vi "sub_ofdm_mes_ce.vi"(11 "ZF channel estimates":cdb[](array[numeric])) -> (3 "interpolated mes carrier CE":cdb[](array[numeric]))   [LabVIEW 2014]
panel:
  out "output size":i32
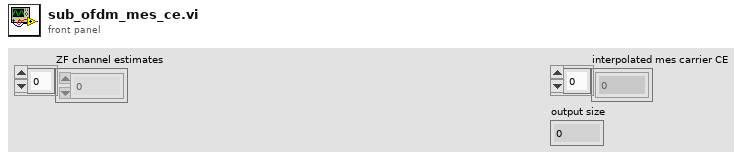
[diagram p1: front panel]
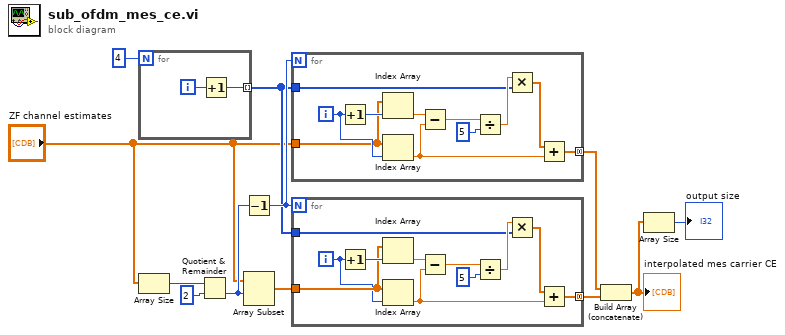
[diagram p0: block diagram]
diagram:
  n1 = for {
    N: 4 -> [_]
    tunnel: [w13] -> w7 mode=indexing
    i -> [w14]
    n2 = Increment(x=w14) -> (x+1=w13:i32)
  }
  n3 = Array Size(array="ZF channel estimates") -> (size(s)=w12:i32)
  n4 = Quotient & Remainder(x=w12, y=2) -> (floor(x/y)=w10:i32)  [unwired: 1 out]
  n5 = Decrement(x=w10) -> (x-1=w9:i32)
  n6 = Array Subset(array="ZF channel estimates", index=w10) -> (w4:cdb[])  [unwired: 1 in]
  n7 = for {
    N: w9 -> [_]
    tunnel: "ZF channel estimates" -> [w23]
    tunnel: w7 -> [w19]
    tunnel: [w17] -> w5 mode=concatenating
    i -> [w24]
    n8 = Increment(x=w24) -> (x+1=w25:i32)
    n9 = Index Array(array=w23, index=w25) -> (element=w15:cdb)
    n10 = Index Array(array=w23, index=w24) -> (element=w16:cdb)
    n11 = Subtract(x=w15, y=w16) -> (x-y=w22:cdb)
    n12 = Divide(x=w22, y=5) -> (x/y=w20:cdb)
    n13 = Multiply(x=w20, y=w19) -> (x*y=w18:cdb[])
    n14 = Add(x=w18, y=w16) -> (x+y=w17:cdb[])
  }
  n15 = for {
    N: w9 -> [_]
    tunnel: w4 -> [w31]
    tunnel: w7 -> [w29]
    tunnel: [w28] -> w2 mode=concatenating
    i -> [w30]
    n16 = Increment(x=w30) -> (x+1=w32:i32)
    n17 = Index Array(array=w31, index=w32) -> (element=w27:cdb)
    n18 = Index Array(array=w31, index=w30) -> (element=w26:cdb)
    n19 = Subtract(x=w27, y=w26) -> (x-y=w33:cdb)
    n20 = Divide(x=w33, y=5) -> (x/y=w35:cdb)
    n21 = Multiply(x=w35, y=w29) -> (x*y=w36:cdb[])
    n22 = Add(x=w36, y=w26) -> (x+y=w28:cdb[])
  }
  n23 = Build Array (concatenate)(w5, w2) -> (w1:cdb[])
  "interpolated mes carrier CE" <- w1
  n24 = Array Size(array=w1) -> (size(s)=→"output size":i32)
